vi "Protocol Write.vi"(8 "error in (no error)":errorcluster, 9 "timeout":i32=10000, 10 "data":u8[](array[numeric]), 11 "protocol layer in":refnum<class "Network Protocol.lvclass">) -> (0 "error out":errorcluster, 1 "timed out?":bool, 3 "protocol layer out":refnum<class "Network Protocol.lvclass">)   [LabVIEW 2017, in "SubVIs.lvlib" / "Network Protocol.lvclass"]
doc: "This provides an interface for writing to a network bus."
uses:
  <vilib>/Modbus/subvis/Protocol/Interfaces/Network Protocol/Network Protocol.lvclass
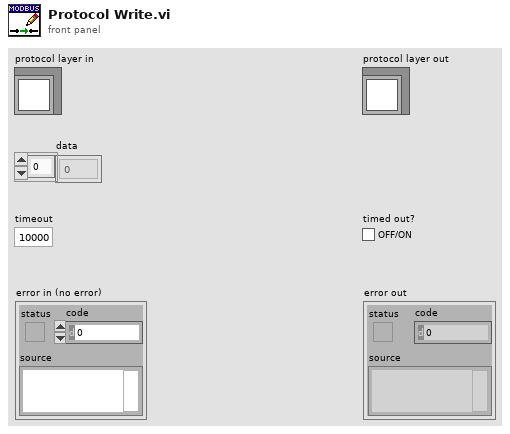
[diagram p1: front panel]
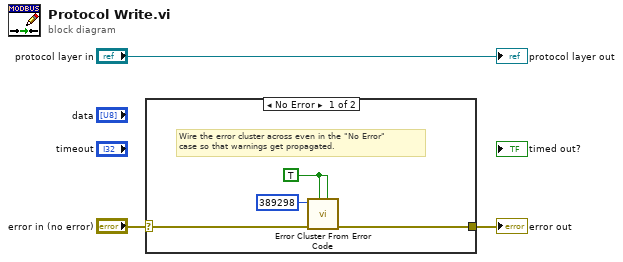
[diagram p0: block diagram]
diagram:
  n1 = case shown="No Error" "error in (no error)" {
    selector: "error in (no error)" -> [w6 w8]
    tunnel: [w7 w8] -> w2
    frame No Error {
      w4 = TRUE ("show call chain? (False)")
      # "Wire the error cluster across even in the \"No Error\"\ncase so that warnings get propagated."
      n2 = call <vilib>:"Error Cluster From Error Code.vi"("is warning? (False)"=w4, "show call chain? (False)"=w4, "error in (no error)"=w6, "error code (0)"=389298) -> ("error out"=w7:errorcluster)  [unwired: 5 in]
    }
    frame Error {
    }
  }
  "error out" <- w2
  "protocol layer out" <- "protocol layer in"
